vi "ALTS-2015 Read Test Type.vi"(8 "error in":errorcluster, 11 "Station Cluster":T1) -> (0 "error out":errorcluster, 3 "Test Type":i32)   [LabVIEW 2013]
uses:
  Controls/ALTS-2015 Station Cluster.ctl
  SLL DAQ Engine/Software/Source Code/Sub VIs/DAQ Engine/Controls/SLL DE List of Digital Inputs.ctl
  SLL DAQ Engine/Software/Source Code/Sub VIs/DAQ Engine/Controls/SLL DE DI Global Options.ctl
  Controls/ALTS-2015 LV2GBL Options.ctl
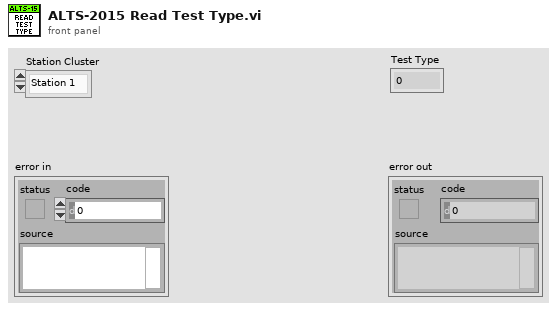
[diagram p1: front panel]
types:
  T1 = typedef "ALTS-2015 Station Cluster.ctl" = enum16{"Station 1", "Station 2", "Station 3", "Station 4"}
  T2 = typedef "ALTS-2015 LV2GBL Options.ctl" = enum16{"Read all", "Write all"}
  T3 = typedef "SLL DE DI Global Options.ctl" = enum16{"Init", "Write Line", "Write Array", "Read Line", "Read Array", "Read Full Status", "Write Full Status"}
  T4 = typedef "SLL DE List of Digital Inputs.ctl" = enum16{"STATION1_START", "STATION1_STOP", "STATION1_CLAMPED", "STATION1_TC_PASS", "STATION1_TC_FAIL", "STATION1_TTA", "STATION1_TTB", "STATION2_START", "STATION2_STOP", "STATION2_CLAMPED", "STATION2_TC_PASS", "STATION2_TC_FAIL", "STATION2_TTA", "STATION2_TTB", "STATION3_START", "STATION3_STOP", "STATION3_CLAMPED", "STATION3_TC_PASS", "STATION3_TC_FAIL", "STATION3_TTA", "STATION3_TTB", "STATION4_START", "STATION4_STOP", "STATION4_CLAMPED", "STATION4_TC_PASS", "STATION4_TC_FAIL", "STATION4_TTA", "STATION4_TTB"}
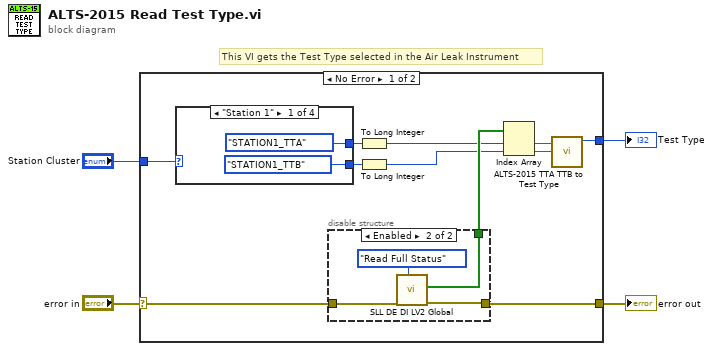
[diagram p0: block diagram]
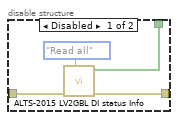
[diagram p2: hidden frame]
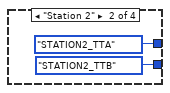
[diagram p3: hidden frame]
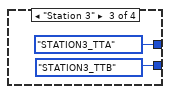
[diagram p4: hidden frame]
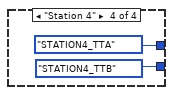
[diagram p5: hidden frame]
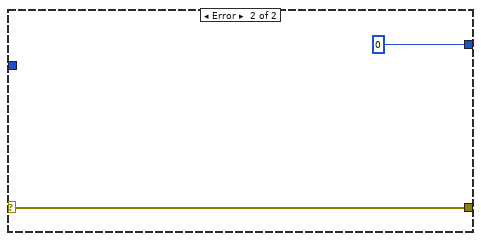
[diagram p6: hidden frame]
diagram:
  # "This VI gets the Test Type selected in the Air Leak Instrument"
  n1 = case shown="No Error" "error in" {
    selector: "error in" -> [w5 w33]
    tunnel: [w8 w33] -> w4
    tunnel: "Station Cluster" -> [w7 _]
    tunnel: [w6 0 ("Test Type")] -> w2
    frame No Error {
      n2 = case shown="\"Station 1\"" w7 {
        tunnel: [SLL_DE_List_of_Digital_Inputs."STATION1_TTA" ("DI Channel Name") SLL_DE_List_of_Digital_Inputs."STATION2_TTA" ("DI Channel Name") SLL_DE_List_of_Digital_Inputs."STATION3_TTA" ("DI Channel Name") SLL_DE_List_of_Digital_Inputs."STATION4_TTA" ("DI Channel Name")] -> w14
        tunnel: [SLL_DE_List_of_Digital_Inputs."STATION1_TTB" ("DI Channel Name") SLL_DE_List_of_Digital_Inputs."STATION2_TTB" ("DI Channel Name") SLL_DE_List_of_Digital_Inputs."STATION3_TTB" ("DI Channel Name") SLL_DE_List_of_Digital_Inputs."STATION4_TTB" ("DI Channel Name")] -> w13
        frame "Station 1" {
        }
        frame "Station 2" {
        }
        frame "Station 3" {
        }
        frame "Station 4" {
        }
      }
      n3 = disable-structure shown="Enabled" {
        disable-tunnel: [w18 w20] -> w15
        disable-tunnel: [w17 w21] -> w8
        disable-tunnel: w5 -> [w16 w22]
        frame Disabled {
          n4 = call "ALTS-2015 LV2GBL DI status Info.vi"("Options"=ALTS-2015_LV2GBL_Options."Read all", "error in"=w16) -> ("error out"=w17:errorcluster, "DI Status Out"=w18:bool[])  [unwired: 8 in]
        }
        frame Enabled {
          n5 = call "SLL DE DI LV2 Global.vi"("Option"=SLL_DE_DI_Global_Options."Read Full Status", "error in (no error)"=w22) -> ("error out"=w21:errorcluster, "Digital Array Status"=w20:bool[])  [unwired: 6 in, 2 out]
        }
      }
      n6 = To Long Integer(number=w14) -> (32bit integer=w12:i32)
      n7 = To Long Integer(number=w13) -> (32bit integer=w11:i32)
      n8 = Index Array(array=w15, index #1=w12, index #2=w11) -> (element #1=w9:bool, element #2=w10:bool)
      n9 = call "ALTS-2015 TTA TTB to Test Type.vi"("TTB"=w10, "TTA"=w9) -> ("Test Type"=w6:i32)  [unwired: 9 in]
    }
    frame Error {
    }
  }
  "error out" <- w4
  "Test Type" <- w2
